vi "Return ID Timeout.vi"(7 "error source vi name":string, 8 "error in (no error)":errorcluster, 10 "id":i32, 11 "ID Pool in":refnum<class "ID Pool.lvclass">) -> (0 "error out":errorcluster, 3 "ID Pool out":refnum<class "ID Pool.lvclass">)   [LabVIEW 2017, in "DSF Core.lvlib" / "ID Pool.lvclass"]
uses:
  ID Pool.lvclass
  Errors.ctl
  <vilib>/NI/Memory Manager/VIs/Source.Write.Scalar.Base10 (I32).vi
  <vilib>/NI/Memory Manager/Static Error Handling.lvlib
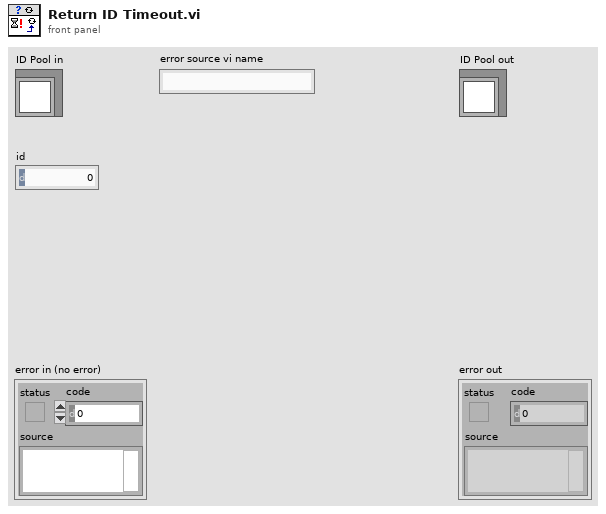
[diagram p1: front panel]
types:
  T1 = typedef "DSF Core.lvlib/ID Pool.lvclass/Errors.ctl" = enum16{"Obtain ID Timeout", "Return ID Timeout"}
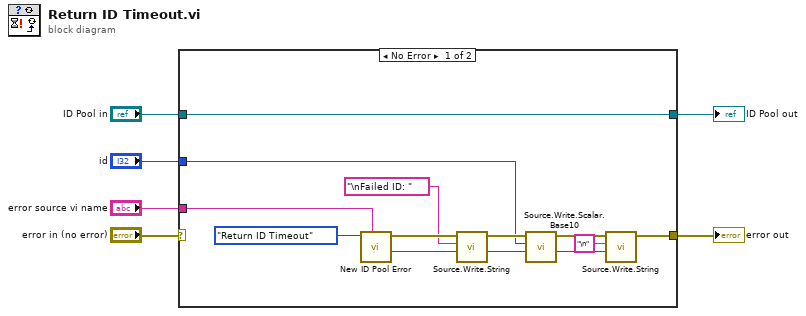
[diagram p0: block diagram]
diagram:
  n1 = case shown="No Error" "error in (no error)" {
    selector: "error in (no error)" -> [_ w20]
    tunnel: "ID Pool in" -> [w19 w21]
    tunnel: [w19 w21] -> w4
    tunnel: [w11 w20] -> w3
    tunnel: "error source vi name" -> [w17 _]
    tunnel: "id" -> [w13 _]
    frame No Error {
      n2 = call "New ID Pool Error.vi"("error source vi name"=w17, "error"=Errors."Return ID Timeout") -> ("new offset"=w9:i32, "error out"=w16:errorcluster)  [unwired: 8 in]
      n3 = call <vilib>:"Source.Write.String.vi"("offset"=w9, "string"="\nFailed ID: ", "error in"=w16) -> ("new offset"=w8:i32, "error out"=w15:errorcluster)  [unwired: 7 in]
      n4 = call-poly <vilib>:"Source.Write.Scalar.Base10.vi"("offset"=w8, "value"=w13, "error in"=w15) -> ("new offset"=w7:i32, "error out"=w12:errorcluster)  [unwired: 7 in]
      n5 = call <vilib>:"Source.Write.String.vi"("offset"=w7, "string"="\n", "error in"=w12) -> ("error out"=w11:errorcluster)  [unwired: 7 in, 1 out]
    }
    frame Error {
    }
  }
  "error out" <- w3
  "ID Pool out" <- w4
